vi "JSONRPC-GetAsString.vi"(10 "index":i32, 11 "params":string[](array[string])) -> (3 "output":string)   [LabVIEW 2013]
uses:
  <vilib>/regexp/Match Regular Expression.xnode
panel:
  # "GetAsString"
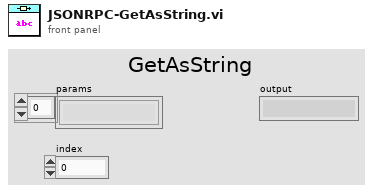
[diagram p1: front panel]
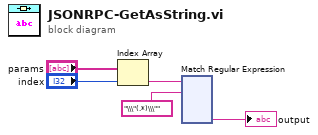
[diagram p0: block diagram]
diagram:
  n1 = Index Array(array="params", index="index") -> (element=w3:string)
  n2 = xnode "Match Regular Expression"("input string"=w3, "regular expression"="\\\"(.*)\\\"") -> ("submatch 1"=→"output":string)  [unwired: 4 in, 5 out]
